vi "Dashboard Main.vi"() -> ()   [LabVIEW 2020]
uses:
  Support/Utility/FP_Size VI to Decoration Simple.vi/TypeDefs_Utility/Cluster_FP Set.ctl
  Support/Utility/FP_Size VI to Decoration Simple.vi/TypeDefs_Utility/ENUM RB_Pos_Quadrant Position.ctl
  <vilib>/event_ctls.llb/eventvkey.ctl
  a666340f-301f-4806-b1ce-2e5969000446.vi
  58c67c19-ca0f-4a2d-b08c-13e7632b1952.vi
  <vilib>/Rock Robotics/Network Tables/NT Read Numeric Array.vi
  <vilib>/Rock Robotics/WPI/Dashboard/WPI_DashboardLogging Global.vi
panel:
  out "Color 2":u32(colorbox)
  in  "Balance Speed":dbl=10.0 min=1.0 max=16.0 step=0.1 format="%.1g"
  out "RIO":string
  out "blink":bool
  out "Heartbeat":dbl
  out "Camera Image Right":T1(plugin-control)
  in  "Auto Select":string(combo)
  in  "Camera Settings Right":T2={"Frame Rate"=30, "Compression"=30, "Size"=1, "DB Camera Config"=FALSE} {"Frame Rate" scale=1.0..30.0; "Compression" scale=100.0..-1.0; "Size" items=["640x480", "320x240", "160x120"]}
  in  "Camera Name Right":string(combo)="No Camera Selection"
  out "Camera Perf":string
  in  "Camera Settings":T2={"Frame Rate"=30, "Compression"=30, "Size"=1, "DB Camera Config"=FALSE} {"Frame Rate" scale=1.0..30.0; "Compression" scale=100.0..-1.0; "Size" items=["640x480", "320x240", "160x120"]}
  in  "TCP":refnum<k5>
  in  "Rec Mode":enum32{"Stop", "Record", "Playback"}(radio)
  out "Robot IP":string
  out "Image Message":string="Timeout in Camera Communications"
  in  "Dashboard Tab":T3(tab)
  out "NT Connection":bool
  out "MotorChart R":cluster{"Numeric":dbl, "Numeric":dbl}(graph)
  out "MotorChart L":cluster{"Numeric":dbl, "Numeric":dbl}(graph)
  out "MotorSliders R":cluster{"MotorSlide1":dbl, "MotorSlide2":dbl} {"MotorSlide2" scale=-1.0..1.0 scale format="%#_2e"; "MotorSlide1" scale=-1.0..1.0 scale format="%#_2e"}
  out "MotorSliders L":cluster{"MotorSlide1":dbl, "MotorSlide2":dbl} {"MotorSlide2" scale=-1.0..1.0 scale format="%#_2e"; "MotorSlide1" scale=-1.0..1.0 scale format="%#_2e"}
  out "Gyro":dbl(knob) scale=0.0..360.0
  out "JS1 Z":dbl(slide) scale=-1.0..1.0 scale format="%#_2e"
  out "JS1 Graph":cluster{"X":dbl, "Y":dbl}[](graph)
  out "JS1 Buttons":T4
  out "JS2 Z":dbl(slide) scale=-1.0..1.0 scale format="%#_2e"
  out "JS2 Graph":cluster{"X":dbl, "Y":dbl}[](graph)
  out "JS2 Buttons":T4
  out "Mode":T5(ring)=enum."Auto Disabled"
  out "Right Camera Perf":cluster{"Bandwidth (Mbps)":dbl, "FPS":dbl}
  in  "DB/String 9":string
  in  "DB/String 8":string
  in  "DB/String 7":string
  in  "DB/String 6":string
  in  "DB/String 5":string
  in  "DB/String 4":string
  in  "DB/String 3":string
  in  "DB/String 2":string
  in  "DB/String 1":string
  in  "DB/String 0":string
  in  "DB/Slider 0":dbl(slide) scale=0.0..5.0
  in  "DB/Slider 1":dbl(slide) scale=0.0..5.0
  in  "DB/Slider 2":dbl(slide) scale=0.0..5.0
  in  "DB/Slider 3":dbl(slide) scale=0.0..5.0
  out "DB/LED 3":bool
  out "DB/LED 2":bool
  out "DB/LED 1":bool
  out "DB/LED 0":bool
  in  "DB/Button 3":bool
  in  "DB/Button 2":bool
  in  "DB/Button 1":bool
  in  "DB/Button 0":bool caption="New Name"
  in  "Test Slider":dbl(slide) scale=0.0..100.0 scale format="%#_3g"
  in  "On/Off":bool caption="Solenoid"
  in  "Test Name":u16(ring) items=["Select the test to run..."]
  in  "Test Tree":string(tree)
  in  "Motor":cluster{"Value":dbl, "Enable":bool} {"Value" scale=-1.0..1.0 scale format="%#_3g"}
  out "Progress":T6 {"Test Progress" scale=0.0..100.0}
  in  "Rev/Fwd":cluster{"Forward":bool, "Reverse":bool}
  in  "Test Ring":u16(ring) items=["Monochrome", "Color"]
  in  "CheckList":i32(listbox)
  out "Tree":string(tree)
  out "Camera Image":T1(plugin-control)
  in  "Camera Name":string(combo)="No Camera Selection"
  # "HW"
  # "HW"
  # "Joysticks"
  # "Drive Motors"
  # "Front"
  # "Right"
  # "Left"
  # "Back"
  # "This tab is a great place for autonomous settings and robot-specific values.\nPlace controls and indicators inside this tab and match name to\nDashboard Variables on robot. You can also delete this comment."
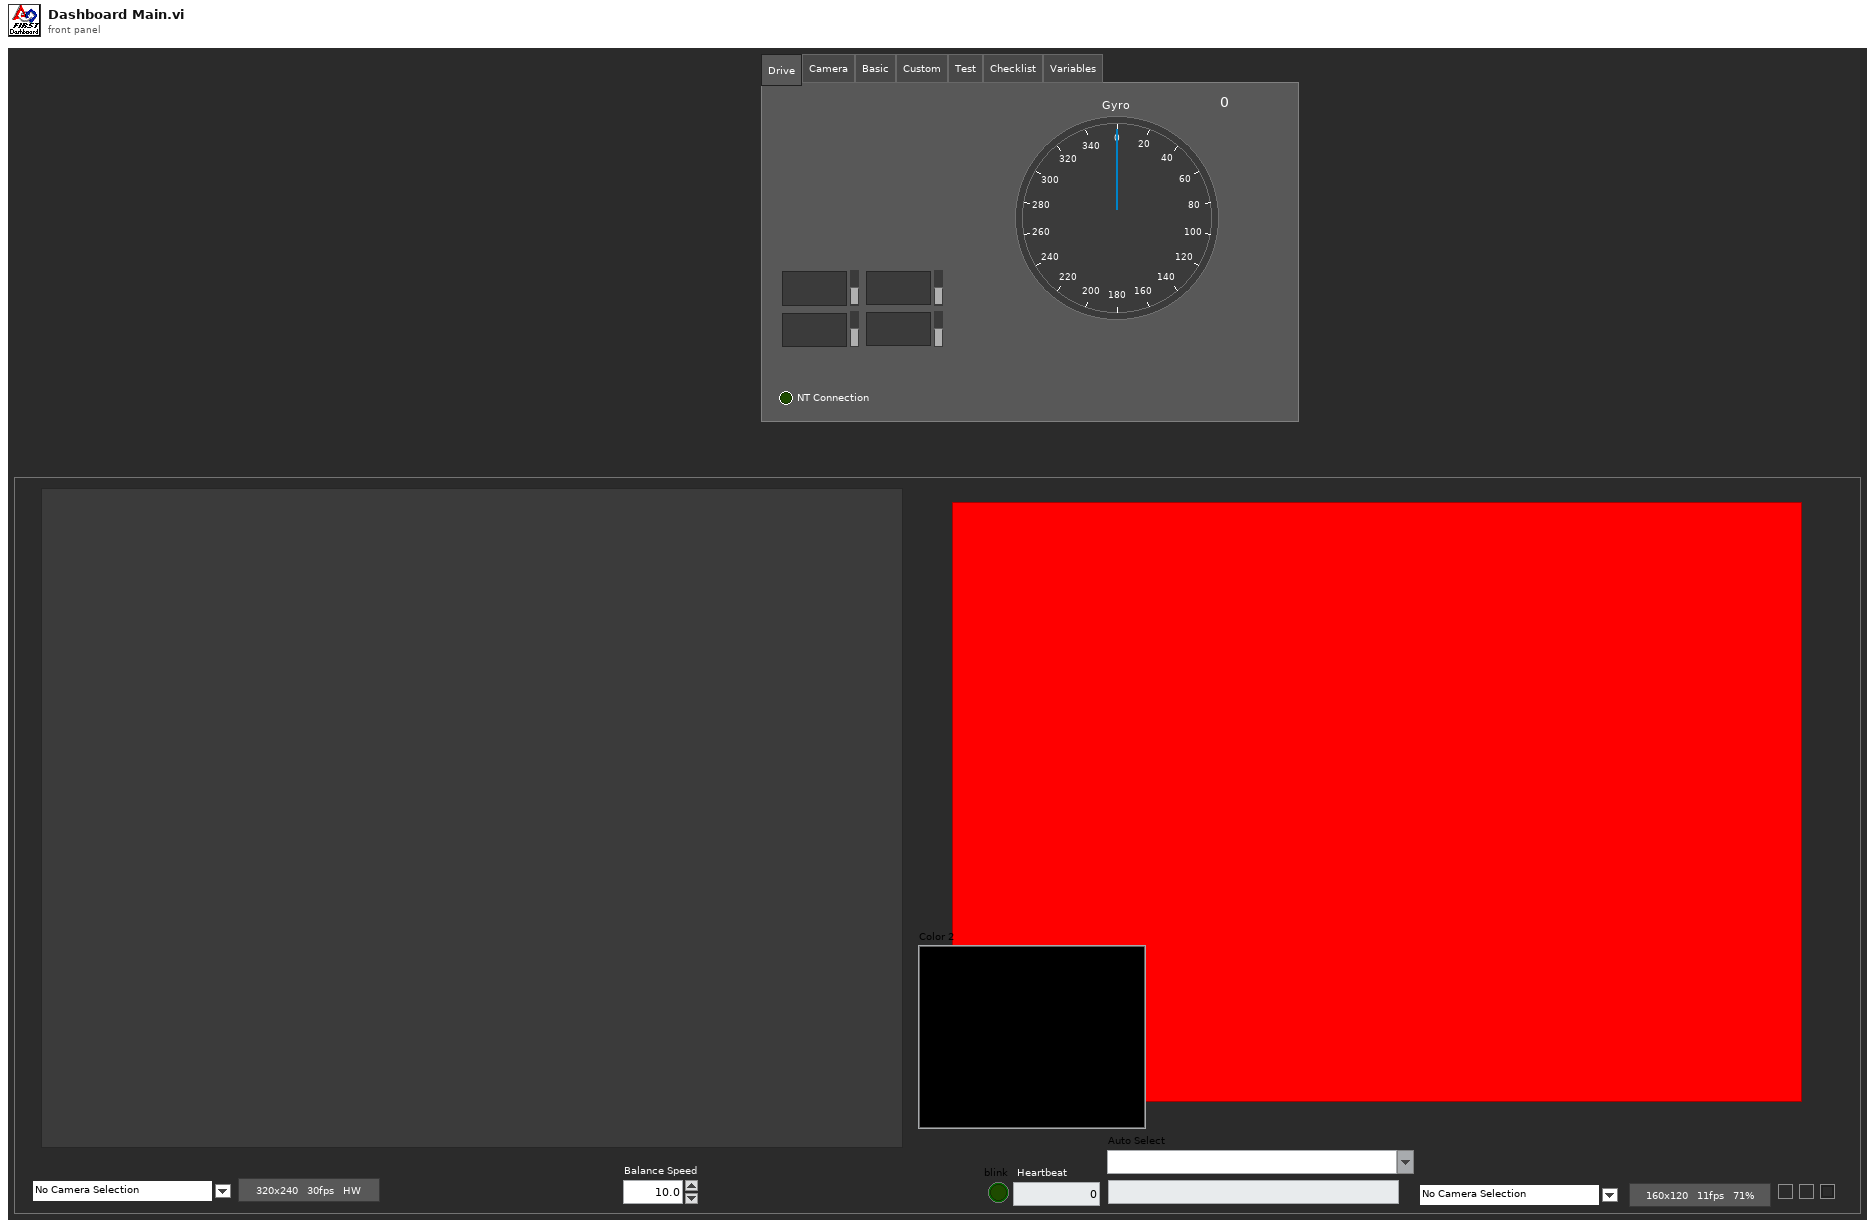
[diagram p1: front panel]
types:
  T1 = typedef "IMAQ Image.ctl" = refnum<image>
  T2 = cluster{"Frame Rate":i32, "Compression":i32, "Size":u16, "DB Camera Config":bool}
  T3 = enum32{"Drive", "Camera", "Basic", "Custom", "Test", "Checklist", "Variables"}
  T4 = cluster{bool, bool, bool, bool, bool, bool, bool, bool, bool, bool, bool, bool}
  T5 = enum8{"Tele-Op Disabled", "Tele-Op Enabled", "Auto Disabled", "Auto Enabled", "Test Disabled", "Test Enabled", "Disconnected", "No Code", "E-Stop"}
  T6 = cluster{"Test Progress":u8, "Test Progress Text":string}
  T7 = cluster{"Save Path":path, "Interval (s)":dbl, "Keep":i32}
  T8 = enum32{"Drive", "Camera", "Basic", "Custom", "Test", "Commands", "Checklist", "Variables"}
  T9 = typedef "Image Type" = u32
  T10 = cluster{"Error Strings":string, "Disable Counts":cluster{u16, u16}, "Rail Faults":cluster{u16, u16, u16}, "Robot IP":string, "DB Mode":u8, "Event Info":cluster{"Name":string, "Type":u8, "Number":u16, "Replay":u8}}
  T11 = cluster{"Storage":cluster{"Disk Free":u64, "RAM Block":u32, "RAM free":u32}, "CPU Utilization":cluster{"CPU % ISR":sgl, "CPU % Time Crit":sgl, "CPU % Timed Str":sgl, "CPU % High":sgl, "CPU % Above":sgl, "CPU % Normal":sgl, "CPU % Low":sgl}, "CAN":cluster{"% Bus Utilization":sgl, "Bus Off Cnt":u32, "TX_FIFO Full Cnt":u32, "Receive Error Cnt":u8, "Transmit Error Cnt":u8}, "HID":cluster{"HID Outputs":u32, "Rumble Low":u16, "Rumble High":u16}[]}
  T12 = cluster{"Status bits":cluster{"Test Mode":bool, "Autonomous":bool, "Enabled":bool, "Code Start":bool, "Brownout":bool, "Reserved 2":bool, "Reserved 3":bool, "E-Stop":bool}, "Code Trace":cluster{"Disabled":bool, "TeleOp":bool, "Auto":bool, "Test":bool}, "Controller Type":enum16{"unknown", "cRIO", "roboRio"}, "Code?":enum16{"unknown", "noCode", "code"}, "Battery V":dbl}
  T13 = cluster{"Control Bits":cluster{"TestMode":bool, "Autonomous":bool, "Enabled":bool, "FMS Present":bool, bool, bool, bool, "E-Stop":bool}, "Team Station ":u8, "Countdown":sgl, "Joystick Values":cluster{"Axes":dbl[], "Buttons":bool[], "POVs":i16[]}[]}
  T14 = cluster{"Axes":dbl[], "Buttons":bool[], "POVs":i16[]}[]
  T15 = cluster{"Axes":dbl[], "Buttons":bool[], "POVs":i16[]}
  T16 = cluster{"Buttons[0]":bool, "Buttons[1]":bool, "Buttons[2]":bool, "Buttons[3]":bool, "Buttons[4]":bool, "Buttons[5]":bool, "Buttons[6]":bool, "Buttons[7]":bool, "Buttons[8]":bool, "Buttons[9]":bool, "Buttons[10]":bool, "Buttons[11]":bool}
  T17 = typedef "Cluster_FP Set.ctl" = cluster{"Menu Bar":bool, "Position":T18, "Decoration index":i32, "border(px)":i32, "Monitor #":i32}
  T18 = typedef "ENUM RB_Pos_Quadrant Position.ctl" = enum32{"LFT-TOP", "MID-TOP", "RGT-TOP", "LFT-CTR", "MID-CTR", "RGT-CTR", "LFT-BOT", "MID-BOT", "RGT-BOT"}
  T19 = cluster{"Camera Image":refnum<vi>, "Tab":refnum<vi>, "Tab Button":refnum<vi>, "Rec Mode":refnum<vi>, "Test Slide":refnum<vi>, "Test On/Off":refnum<vi>, "Test Ring":refnum<vi>, "Test R/F":refnum<vi>, "Test Name":refnum<vi>, "Motor":refnum<vi>, "Progress":refnum<vi>, "LstBox Refnum":refnum<vi>, "Test Tree":refnum<vi>, "VblTree":refnum<vi>, "Camera Settings":refnum<vi>, "Camera Name":refnum<vi>, "perf info":refnum<vi>, "Camera Settings 2":refnum<vi>, "Camera Name 2":refnum<vi>, "Image Right":refnum<vi>}
  T20 = cluster{"Global Rectangle":i32[], "Contours":cluster{"Contour Type":u32, "ROI Type":u32, "Points":i32[]}[]}
  T21 = cluster{"Camera Name":string, string, "Saved DB Images Info":cluster{"Save Path":path, "Interval (s)":dbl, "Keep":i32}}
  T22 = cluster{"Camera Name Right":string, string, "Saved DB Images Info":cluster{"Save Path":path, "Interval (s)":dbl, "Keep":i32}}
  T23 = cluster{"Operation":enum16{"Update", "Clear"}, "Color Box":u32}[]
  T24 = typedef "eventvkey.ctl" = enum16{"ASCII", "Enter", "Return", "Shift", "Ctrl", "Alt", "Cmd", "Opt", "Caps", "NumLock", "Clear", "Break", "Up", "Down", "Left", "Right", "Insert", "Delete", "Home", "End", "PageUp", "PageDown", "Escape", "Help", "Pause", "ScrollLock", "F1", "F2", "F3", "F4", "F5", "F6", "F7", "F8", "F9", "F10", "F11", "F12", "F13", "F14", "F15", "F16", "F17", "F18", "F19", "F20", "F21", "F22", "F23", "F24", "Play", "VolumeUp", "VolumeDown", "Mute", "Two Byte Char"}
  T25 = cluster{"Image Size":bool, "Image Type":bool, "Pixel Value":bool, "ROI Information":bool, "Zoom Factor":bool}
  T26 = cluster{"Operation":enum16{"Update", "Clear"}, "Color Box":u32}
  T27 = cluster{"Shift":bool, "Ctrl":bool, "Alt":bool, "Cmd":bool, "Opt":bool}
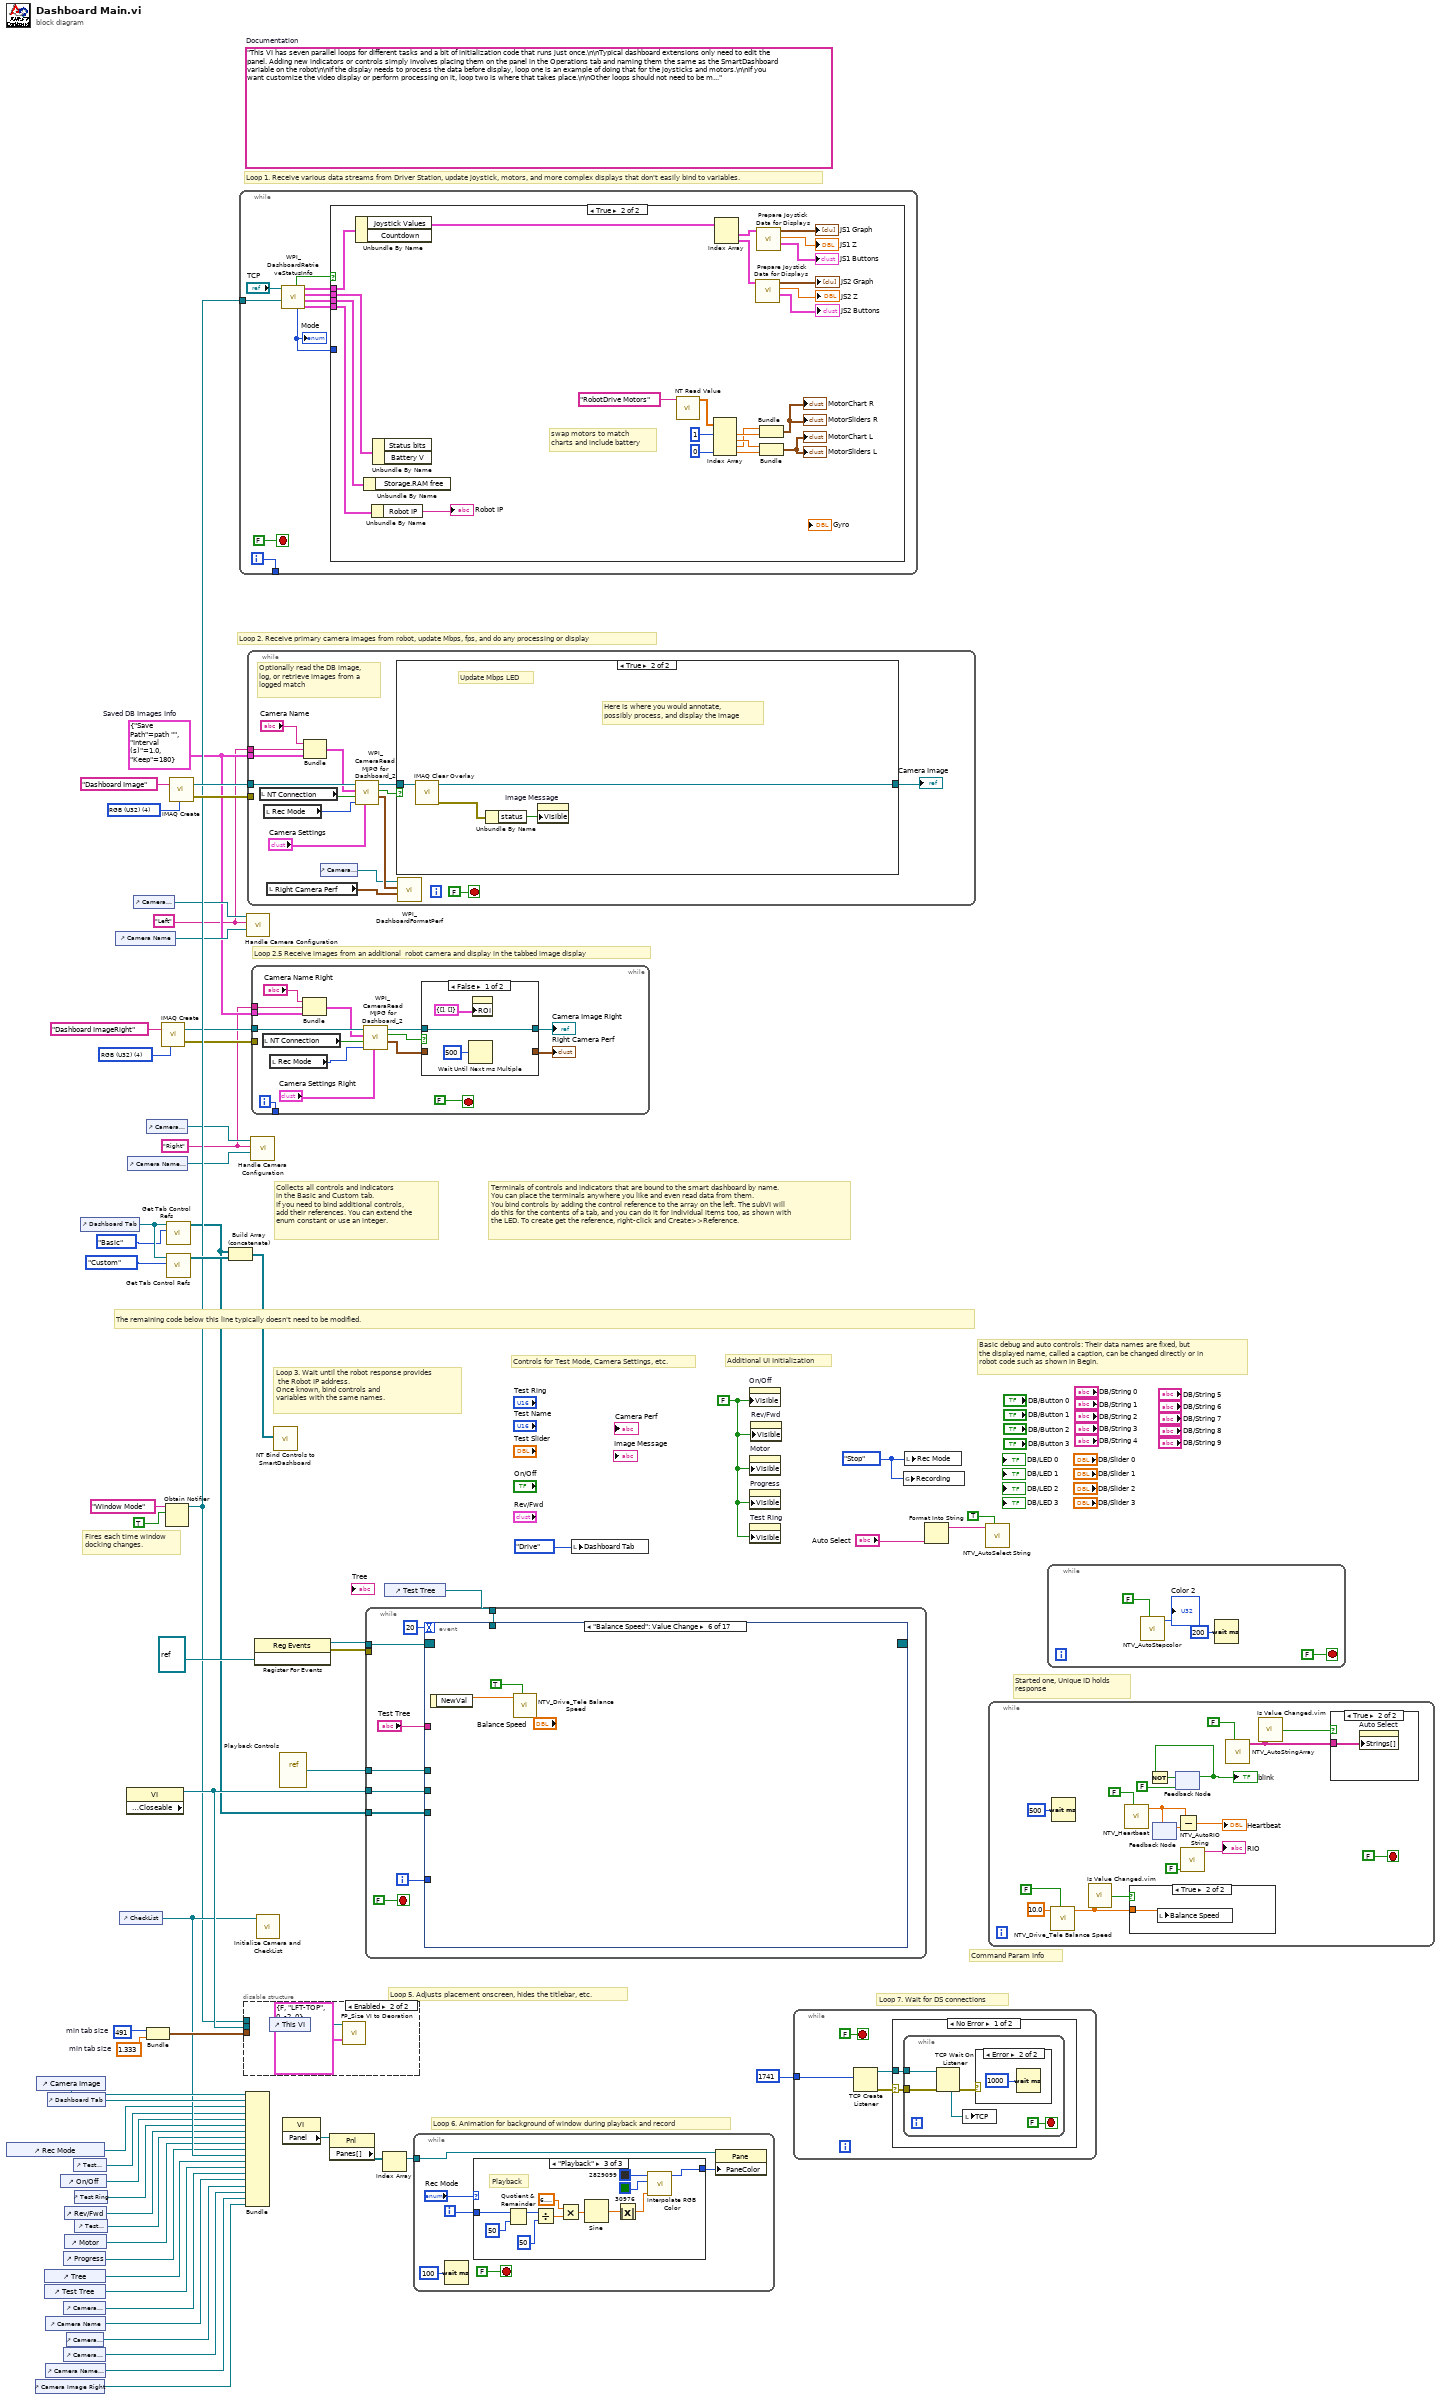
[diagram p0: block diagram]
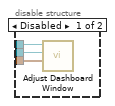
[diagram p4: hidden frame]
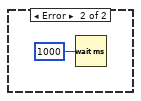
[diagram p7: hidden frame]
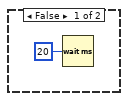
[diagram p8: hidden frame]
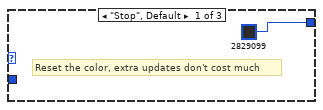
[diagram p9: hidden frame]
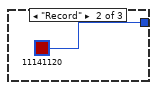
[diagram p10: hidden frame]
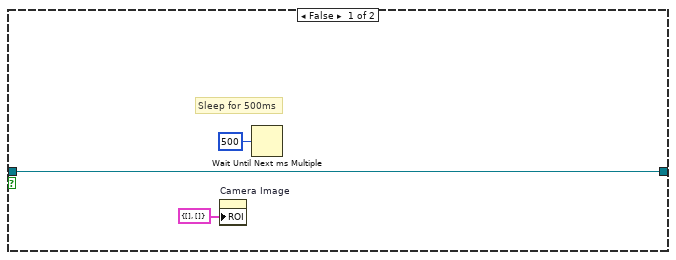
[diagram p11: hidden frame]
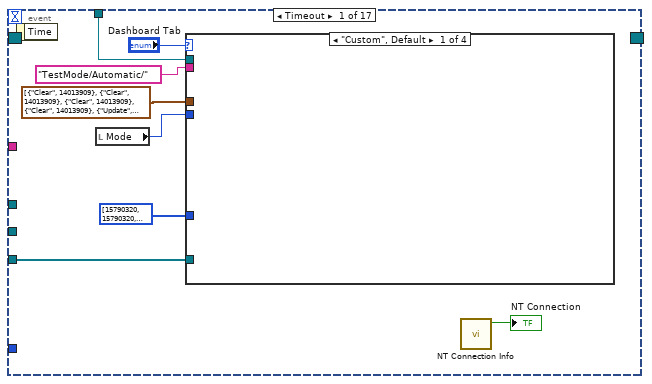
[diagram p12: hidden frame]
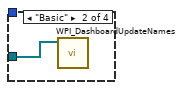
[diagram p13: hidden frame]
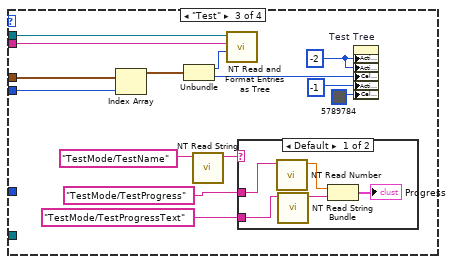
[diagram p14: hidden frame]
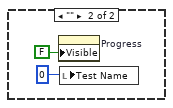
[diagram p15: hidden frame]
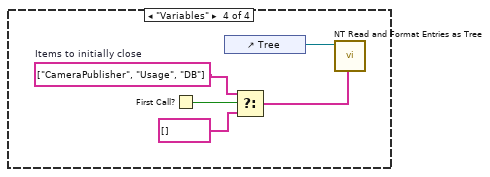
[diagram p16: hidden frame]
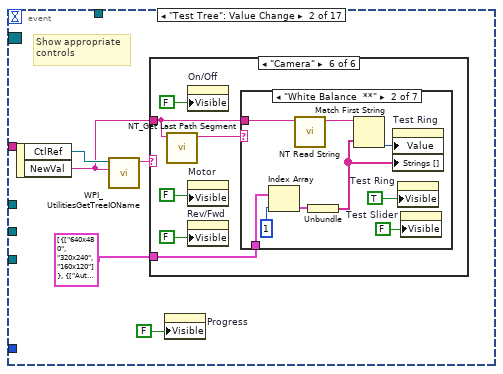
[diagram p17: hidden frame]
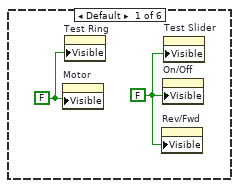
[diagram p18: hidden frame]
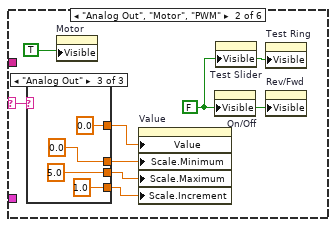
[diagram p19: hidden frame]
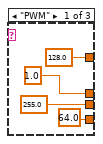
[diagram p20: hidden frame]
diagram:
  w6 = T7 {"Save Path"=path "", "Interval (s)"=1.0, "Keep"=180}  # Saved DB Images Info
  w5 = "Right"
  w4 = "Left"
  w16 = T9 4 items=["Grayscale (U8)", "Grayscale (I16)", "Grayscale (SGL)", "Complex (CSG)", "RGB (U32)", "HSL (U32)", "RGB (U64)"] ("Image Type")
  w41 = 491  # min tab size
  w40 = 1.333  # min tab size
  w48 = enum32{"Stop", "Record", "Playback"}."Stop" ("Rec Mode")
  w27 = FALSE ("Visible")
  (unwired) "This VI has seven parallel loops for different tasks and a bit of initialization code that runs just once.\n\nTypical dashboard extensions only need to edit the panel. Adding new indicators or controls simply involves placing them on the panel in the Operations tab and naming them the same as the SmartDashboard variable on the robot\n\nIf the display needs to process the data before display, loop one is an example of doing that for the joysticks and motors.\n\nIf you want customize the video display or perform processing on it, loop two is where that takes place.\n\nOther loops should not need to be modified. They are pretty standard, and document the task they perform."  # Documentation
  w62 = T9 4 items=["Grayscale (U8)", "Grayscale (I16)", "Grayscale (SGL)", "Complex (CSG)", "RGB (U32)", "HSL (U32)", "RGB (U64)"] ("Image Type")
  # "Loop 2.5 Receive images from an additional  robot camera and display in the tabbed image display"
  # "Command Param Info"
  # "Started one, Unique ID holds\nresponse"
  # "Loop 7. Wait for DS connections"
  # "Basic debug and auto controls: Their data names are fixed, but\nthe displayed name, called a caption, can be changed directly or in\nrobot code such as shown in Begin."
  # "Controls for Test Mode, Camera Settings, etc."
  # "Additional UI Initialization"
  # "Loop 6. Animation for background of window during playback and record"
  # "Fires each time window\ndocking changes."
  # "Collects all controls and indicators\nin the Basic and Custom tab.\nIf you need to bind additional controls,\nadd their references. You can extend the\nenum constant or use an integer."
  # "The remaining code below this line typically doesn't need to be modified."
  # "Terminals of controls and indicators that are bound to the smart dashboard by name.\nYou can place the terminals anywhere you like and even read data from them.\nYou bind controls by adding the control reference to the array on the left. The subVI will\ndo this for the contents of a tab, and you can do it for individual items too, as shown with\nthe LED. To create get the reference, right-click and Create>>Reference."
  # "Loop 3. Wait until the robot response provides\n the Robot IP address.\nOnce known, bind controls and\nvariables with the same names."
  # "Loop 5. Adjusts placement onscreen, hides the titlebar, etc."
  # "Loop 1. Receive various data streams from Driver Station, update joystick, motors, and more complex displays that don't easily bind to variables."
  # "Loop 2. Receive primary camera images from robot, update Mbps, fps, and do any processing or display"
  n1 = control-ref of="Rec Mode"() -> (w33:refnum<vi>)
  n2 = control-ref of="Camera Image Right"() -> (w9:refnum<vi>)
  n3 = control-ref of="Camera Image"() -> (w43:refnum<vi>)
  n4 = control-ref of="Tree"() -> (w37:refnum<vi>)
  n5 = control-ref of="Test Tree"() -> (w36:refnum<vi>)
  n6 = control-ref of="Camera Name"() -> (w20:refnum<vi>)
  n7 = control-ref of="Camera Name Right"() -> (w10:refnum<vi>)
  n8 = control-ref of="Dashboard Tab"() -> (w42:refnum<vi>)
  n9 = control-ref of="On/Off"() -> (w31:refnum<vi>)
  n10 = control-ref of="Progress"() -> (w28:refnum<vi>)
  n11 = control-ref of="Camera Settings"() -> (w21:refnum<vi>)
  n12 = control-ref of="Camera Settings Right"() -> (w11:refnum<vi>)
  n13 = control-ref of="Rev/Fwd"() -> (w29:refnum<vi>)
  n14 = control-ref of="Motor"() -> (w34:refnum<vi>)
  n15 = control-ref of="Camera Perf"() -> (w19:refnum<vi>)
  n16 = control-ref of="Test Slider"() -> (w32:refnum<vi>)
  n17 = control-ref of="Test Ring"() -> (w30:refnum<vi>)
  n18 = control-ref of="Test Name"() -> (w35:refnum<vi>)
  n19 = control-ref of="Dashboard Tab"() -> (w46:refnum<vi>)
  n20 = control-ref of="Camera Name"() -> (w22:refnum<vi>)
  n21 = control-ref of="CheckList"() -> (w38:refnum<vi>)
  n22 = property class="VI" props=["Front Panel.Closeable"]() -> (reference out=w47:refnum<vi>)  [unwired: 2 in, 2 out]
  n23 = control-ref of="Camera Name Right"() -> (w12:refnum<vi>)
  n24 = control-ref of="Camera Settings"() -> (w23:refnum<vi>)
  n25 = control-ref of="Camera Settings Right"() -> (w13:refnum<vi>)
  n26 = Bundle("min tab size"=w41, "min tab size"=w40) -> (w39:cluster{"min tab size":i32, "min tab size":dbl})  [unwired: 1 in]
  n27 = call "IMAQ Create"("Image Name"="Dashboard ImageRight", "Image Type"=w16) -> ("New Image"=w15:T1, "error out"=w14:errorcluster)  [unwired: 2 in, 1 out]
  n28 = Obtain Notifier(name (unnamed)="Window Mode", notification data type=TRUE) -> (notifier out=w26:refnum<notifier>)  [unwired: 2 in, 2 out]
  n29 = call <vilib>:"Get Tab Control Refs.vi"("Page Index"=T8."Basic" ("Dashboard Tab"), "TabControl in"=w46) -> ("ControlsOnPage"=w18:refnum<vi>[])  [unwired: 9 in]
  n30 = call <vilib>:"Get Tab Control Refs.vi"("Page Index"=T8."Custom" ("Dashboard Tab"), "TabControl in"=w46) -> ("ControlsOnPage"=w45:refnum<vi>[])  [unwired: 9 in]
  n31 = call "IMAQ Create"("Image Name"="Dashboard Image", "Image Type"=w62) -> ("New Image"=w60:T1, "error out"=w59:errorcluster)  [unwired: 2 in, 1 out]
  n32 = Build Array (concatenate)(w18, w45) -> (w44:refnum<vi>[])
  n33 = while {
    tunnel: [w71] -> _
    tunnel: w26 -> [w63]
    i -> [w71]
    stop <- FALSE stop-if-true
    n34 = call <vilib>:"WPI_DashboardRetrieveStatusInfo.vi"("Window Mode Notifier"=w63, "TCP Cnx"="TCP") -> ("Power and Errors"=w66:T10, "Robot Metrics"=w69:T11, "Status Info"=w70:T12, "Control Info"=w67:T13, "Robot Mode"=w65:T5, "Process?"=w68:bool)  [unwired: 4 in]
    "Mode" <- w65
    n35 = case shown="True" w68 {
      tunnel: w70 -> [_ w97]
      tunnel: w69 -> [_ w96]
      tunnel: w67 -> [_ w95]
      tunnel: w66 -> [_ w94]
      tunnel: w65 -> [_ _]
      frame False {
        n36 = Wait (ms)(milliseconds to wait=u32 20) -> ()  [unwired: 1 out]
      }
      frame True {
        # "swap motors to match\ncharts and include battery"
        n37 = Unbundle By Name(w95) -> ("Joystick Values"=w85:T14)  [unwired: 1 out]
        n38 = Unbundle By Name(w96) -> ()  [unwired: 1 out]
        n39 = Unbundle By Name(w94) -> ("Robot IP"=→"Robot IP":string)
        n40 = Unbundle By Name(w97) -> ()  [unwired: 2 out]
        n41 = call-poly <vilib>:"NT Read Value.vi"("name"="RobotDrive Motors" ("Name")) -> ("value"=w75:dbl[])  [unwired: 8 in, 2 out]
        n42 = Index Array(array=w75, index #1=1, index #4=0) -> (element #1=w89:dbl, element #2=w90:dbl, element #3=w88:dbl, element #4=w93:dbl)  [unwired: 2 in]
        n43 = Index Array(array=w85) -> (element #1=w84:T15, element #2=w80:T15)  [unwired: 2 in]
        n44 = call "Prepare Joystick Data for Displays.vi"("Joystick Values"=w80) -> ("Buttons"=→"JS2 Buttons":T16, "Z Axis"=→"JS2 Z":dbl, "Cartesian Data"=→"JS2 Graph":cluster{"X axis":dbl, "X axis":dbl}[])  [unwired: 8 in]
        n45 = call "Prepare Joystick Data for Displays.vi"("Joystick Values"=w84) -> ("Buttons"=→"JS1 Buttons":T16, "Z Axis"=→"JS1 Z":dbl, "Cartesian Data"=→"JS1 Graph":cluster{"X axis":dbl, "X axis":dbl}[])  [unwired: 8 in]
        n46 = Bundle("Numeric"=w88, "Numeric"=w89) -> (→"MotorChart R" →"MotorSliders R":cluster{"Numeric":dbl, "Numeric":dbl})  [unwired: 1 in]
        n47 = Bundle("Numeric"=w90, "Numeric"=w93) -> (→"MotorChart L" →"MotorSliders L":cluster{"Numeric":dbl, "Numeric":dbl})  [unwired: 1 in]
      }
    }
  }
  n48 = disable-structure shown="Enabled" {
    disable-tunnel: w47 -> [w101 _]
    disable-tunnel: w39 -> [w100 _]
    disable-tunnel: w26 -> [w98 _]
    frame Disabled {
      n49 = call "Adjust Dashboard Window.vi"("Size Constraints"=w100, "VI"=w101, "WIn Mode"=w98) -> ("Sizing Refnums"=w99:T19)  [unwired: 8 in]
    }
    frame Enabled {
      n50 = control-ref of="This VI"() -> (w103:refnum<vi>)
      n51 = call "FP_Size VI to Deoration.vi"("FPSet"=T17 {"Menu Bar"=FALSE, "Position"=enum."LFT-TOP", "Decoration index"=0, "border(px)"=-2, "Monitor #"=0}, "VI Ref"=w103) -> ()  [unwired: 8 in, 2 out]
    }
  }
  n52 = Bundle("Camera Image"=w43, "Dashboard Tab"=w42, "Rec Mode"=w33, "Test Slider"=w32, "On/Off"=w31, "Test Ring"=w30, "Rev/Fwd"=w29, "Test Name"=w35, "Motor"=w34, "Progress"=w28, "CheckList"=w38, "Tree"=w37, "Test Tree"=w36, "Camera Settings"=w21, "Camera Name"=w20, "Camera Perf"=w19, "Camera Settings Right"=w11, "Camera Name Right"=w10, "Camera Image Right"=w9) -> ()  [unwired: 1 in, 1 out]
  n53 = call "Handle Camera Configuration.vi"("CameraNameRef"=w22, "Display Name"=w4, "ClusterRef"=w23) -> ()  [unwired: 9 in]
  n54 = while {
    tunnel: w60 -> [w117]
    tunnel: w59 -> [_]
    tunnel: w6 -> [w110]
    tunnel: w4 -> [w107]
    stop <- FALSE stop-if-true
    # "Optionally read the DB image,\nlog, or retrieve images from a\nlogged match"
    n55 = local read "NT Connection"() -> (w111:bool)
    n56 = local read "Rec Mode"() -> (w114:enum32{"Stop", "Record", "Playback"})
    n57 = local read "Right Camera Perf"() -> (w105:cluster{"Bandwidth (Mbps)":dbl, "FPS":dbl})
    n58 = Bundle("Camera Name"="Camera Name", w107, "Saved DB Images Info"=w110) -> (w109:T21)  [unwired: 1 in]
    n59 = control-ref of="Camera Perf"() -> (w104:refnum<vi>)
    n60 = call <vilib>:"WPI_CameraRead MJPG for Dashboard_2.vi"("Camera Settings"="Camera Settings", "Rec Mode"=w114, "NT Connection"=w111, "Capture Info"=w109, "Image in"=w117) -> ("perf info"=w106:cluster{"Bandwidth (Mbps)":dbl, "fps":dbl}, "Active"=w115:bool, "Image\\ out"=w116:T1)  [unwired: 4 in]
    n61 = case shown="True" w115 {
      tunnel: w116 -> [w120 w123]
      tunnel: [w120 w122] -> w112
      frame False {
        # "Sleep for 500ms"
        n62 = property on="Camera Image" class="ImageControl"("ROI"=T20 {"Global Rectangle"=[], "Contours"=[]}) -> ()  [unwired: 2 in, 2 out]
        n63 = Wait Until Next ms Multiple(millisecond multiple=u32 500) -> ()  [unwired: 1 out]
      }
      frame True {
        # "Here is where you would annotate,\npossibly process, and display the image"
        # "Update Mbps LED"
        n64 = call "IMAQ Clear Overlay"("Image"=w123) -> ("error out"=w124:errorcluster, "Image Out"=w122:T1)  [unwired: 2 in, 7 out]
        n65 = Unbundle By Name(w124) -> ("status"=w125:bool)
        n66 = property on="Image Message" class="Str"("Visible"=w125) -> ()  [unwired: 2 in, 2 out]
      }
    }
    "Camera Image" <- w112
    n67 = call <vilib>:"WPI_DashboardFormatPerf.vi"("Right Camera Perf"=w105, "Performance"=w106, "String in"=w104) -> ()  [unwired: 9 in]
  }
  n68 = call "Handle Camera Configuration.vi"("CameraNameRef"=w12, "Display Name"=w5, "ClusterRef"=w13) -> ()  [unwired: 9 in]
  n69 = while {
    tunnel: w15 -> [w140]
    tunnel: w14 -> [_]
    tunnel: [w135] -> _
    tunnel: w6 -> [w131]
    tunnel: w5 -> [w128]
    i -> [w135]
    stop <- FALSE stop-if-true
    n70 = local read "NT Connection"() -> (w132:bool)
    n71 = local read "Rec Mode"() -> (w139:enum32{"Stop", "Record", "Playback"})
    n72 = Bundle("Camera Name Right"="Camera Name Right", w128, "Saved DB Images Info"=w131) -> (w130:T22)  [unwired: 1 in]
    n73 = call <vilib>:"WPI_CameraRead MJPG for Dashboard_2.vi"("Camera Settings"="Camera Settings Right", "Rec Mode"=w139, "NT Connection"=w132, "Capture Info"=w130, "Image in"=w140) -> ("perf info"=w126:cluster{"Bandwidth (Mbps)":dbl, "fps":dbl}, "Active"=w134:bool, "Image\\ out"=w137:T1)  [unwired: 4 in]
    n74 = case shown="False" w134 {
      tunnel: w137 -> [w142 w145]
      tunnel: [w142 w145] -> w133
      tunnel: [_ w144] -> w127
      tunnel: w126 -> [_ w144]
      frame False {
        n75 = Wait Until Next ms Multiple(millisecond multiple=u32 500) -> ()  [unwired: 1 out]
        n76 = property on="Camera Image Right" class="ImageControl"("ROI"=T20 {"Global Rectangle"=[], "Contours"=[]}) -> ()  [unwired: 2 in, 2 out]
      }
      frame True {
      }
    }
    "Camera Image Right" <- w133
    "Right Camera Perf" <- w127
  }
  n77 = register-events(refnum<vi> refnum) -> (reference out=w51:refnum<event-registration>, error out=w50:errorcluster)  [unwired: 2 in]
  n78 = call "Initialize Camera and CheckList.vi"("ListBox in"=w38) -> ()  [unwired: 11 in]
  n79 = call <vilib>:"NT Bind Controls to SmartDashboard.vi"("Bound Control Refs"=w44) -> ()  [unwired: 11 in]
  n80 = vi-ref "Playback Controls.vi"() -> (w52:refnum<vi>)
  n81 = property class="VI"() -> ("Panel"=w54:refnum<vi>)  [unwired: 2 in, 2 out]
  n82 = property class="Pnl"(reference=w54) -> ("Panes[]"=w55:refnum<vi>[])  [unwired: 1 in, 2 out]
  n83 = Index Array(array=w55) -> (element=w53:refnum<vi>)  [unwired: 1 in]
  n84 = control-ref of="Test Tree"() -> (w56:refnum<vi>)
  n85 = while {
    tunnel: w56 -> [w152]
    tunnel: w52 -> [w151]
    tunnel: w51 -> [w150]
    tunnel: w50 -> [_]
    tunnel: w47 -> [w149]
    tunnel: w18 -> [w148]
    i -> [w146]
    stop <- FALSE stop-if-true
    n86 = event shown="[5] \"Balance Speed\": Value Change" {
      selector: w150 -> [_ _ _ _ _ _ _ _ _ _ _ _ _ _ _ _ _]
      dyn-events: [_ _ _ _ _ _ _ _ _ _ _ _ _ w356 _ _ _] -> _
      timeout: 20 -> [_ _ _ _ _ _ _ _ _ _ _ _ _ _ _ _ _]
      tunnel: w152 -> [w161 _ _ _ _ _ _ _ _ _ _ _ _ _ _ _ _]
      tunnel: "Test Tree" -> [_ _ _ _ _ _ _ _ w329 w336 w337 w340 w347 _ _ _ _]
      tunnel: w151 -> [_ _ _ _ _ _ _ _ _ _ _ _ _ w358 _ w373 _]
      tunnel: w149 -> [_ _ _ _ _ _ _ _ _ _ _ _ _ w354 _ _ _]
      tunnel: w148 -> [w156 _ _ _ _ _ _ _ _ _ _ _ _ _ _ _ _]
      tunnel: w146 -> [_ _ _ _ _ _ _ _ _ _ _ _ _ _ _ _ _]
      event Timeout {
        n87 = event-data() -> ()  [unwired: 1 in, 1 out]
        n88 = local read "Mode"() -> (w159:T5)
        n89 = case shown="\"Custom\", Default" "Dashboard Tab" {
          tunnel: w161 -> [_ _ w177 _]
          tunnel: "TestMode/Automatic/" ("Name Pattern") -> [_ _ w176 _]
          tunnel: T23 [{"Operation"=enum."Clear", "Color Box"=14013909}, {"Operation"=enum."Clear", "Color Box"=14013909}, {"Operation"=enum."Clear", "Color Box"=14013909}, {"Operation"=enum."Clear", "Color Box"=14013909}, {"Operation"=enum."Update", "Color Box"=14013909}, {"Operation"=enum."Update", "Color Box"=16777215}, {"Operation"=enum."Clear", "Color Box"=14013909}, {"Operation"=enum."Clear", "Color Box"=14013909}, {"Operation"=enum."Clear", "Color Box"=14013909}] -> [_ _ w169 _]
          tunnel: w159 -> [_ _ w168 _]
          tunnel: u32[] [15790320, 15790320, 15790320, 15790320, 16777215, 16777215, 15790320, 15790320, 15790320] -> [_ _ _ _]
          tunnel: w156 -> [_ w163 _ _]
          frame "Custom", Default {
          }
          frame "Basic" {
            n90 = call <vilib>:"WPI_DashboardUpdateNames.vi"("Controls on Tab"=w163) -> ()  [unwired: 11 in]
          }
          frame "Test" {
            w175 = -2 ("Active Item:Row Number")
            n91 = Index Array(array=w169, index=w168) -> (element=w170:T26)
            n92 = Unbundle(w170) -> ("Operation"=w171:enum16{"Update", "Clear"}, "Color Box"=w172:u32)
            n93 = call <vilib>:"NT Read String.vi"("name"="TestMode/TestName" ("Name")) -> ("value"=w166:string)  [unwired: 8 in, 2 out]
            n94 = call <vilib>:"NT Read and Format Entries as Tree.vi"("Operation"=w171, "Name Pattern"=w176, "Tree Refnum"=w177) -> ()  [unwired: 7 in, 2 out]
            n95 = case shown="Default" w166 {
              tunnel: "TestMode/TestProgress" ("Name") -> [w179 _]
              tunnel: "TestMode/TestProgressText" ("Name") -> [w178 _]
              frame Default {
                n96 = call <vilib>:"NT Read Number.vi"("name"=w179) -> ("value"=w180:dbl)  [unwired: 8 in, 2 out]
                n97 = call <vilib>:"NT Read String.vi"("name"=w178) -> ("value"=w181:string)  [unwired: 8 in, 2 out]
                n98 = Bundle("value"=w180, "value"=w181) -> (→"Progress":cluster{"value":dbl, "value":string})  [unwired: 1 in]
              }
              frame "" {
                n99 = property on="Progress" class="Clust (strict)"("Visible"=FALSE) -> ()  [unwired: 2 in, 2 out]
                n100 = local write "Test Name"(u16 0) -> ()
              }
            }
            n101 = property on="Test Tree" class="Tree (strict)"("Active Item Row Number"=w175, "ActiveColNum"=w175, "CellBG"=w172, "Active Item Row Number"=-1 ("Active Item:Row Number"), "CellBG"=u32 5789784 ("Color Box")) -> ()  [unwired: 2 in, 2 out]
          }
          frame "Variables" {
            w187 = string[] ["CameraPublisher", "Usage", "DB"]  # Items to initially close
            n102 = First Call?() -> (First Call?: T/F=w188:bool)
            n103 = control-ref of="Tree"() -> (w189:refnum<vi>)
            n104 = Select(t=w187, s=w188, f=string[] []) -> (s? t:f=w185:string[])
            n105 = call <vilib>:"NT Read and Format Entries as Tree.vi"("Tags to  Close"=w185, "Tree Refnum"=w189) -> ()  [unwired: 8 in, 2 out]
          }
        }
        n106 = call <vilib>:"NT Connection Info.vi"() -> ("Connected"=→"NT Connection":bool)  [unwired: 11 in]
      }
      event "Test Tree": Value Change {
        # "Show appropriate\ncontrols"
        n107 = event-data() -> ("CtlRef"=w193:refnum<vi>, "NewVal"=w191:string)  [unwired: 1 in]
        n108 = call <vilib>:"WPI_UtilitiesGetTreeIOName.vi"("NewVal"=w191, "TreeControl in"=w193) -> ("I/O Name"=w194:string)  [unwired: 9 in]
        n109 = case shown="\"Camera\"" w194 {
          selector: w194 -> [_ w201 _ w223 w232 _]
          tunnel: w191 -> [_ _ w220 w222 _ w239]
          tunnel: cluster{string[]}[] [{["640x480", "320x240", "160x120"]}, {["Auto", "Fixed indoor", "Fixed outdoor 1", "Fixed outdoor 2", "Fixed fluorescent 1", "Fixed fluorescent 2", "Hold current"]}, {["Auto", "Flicker-free 50 Hz", "Flicker-free 60 Hz", "Hold current"]}, {["None", "Prioritize frame rate", "Prioritize image quality"]}, {["Monochrome", "Color"]}] -> [_ _ _ _ _ w238]
          frame Default {
            w196 = FALSE ("Visible")
            w195 = FALSE ("Visible")
            n110 = property on="Motor" class="Clust (strict)"("Visible"=w195) -> ()  [unwired: 2 in, 2 out]
            n111 = property on="Test Ring" class="Ring (strict)"("Visible"=w195) -> ()  [unwired: 2 in, 2 out]
            n112 = property on="Rev/Fwd" class="Clust (strict)"("Visible"=w196) -> ()  [unwired: 2 in, 2 out]
            n113 = property on="On/Off" class="Bool (strict)"("Visible"=w196) -> ()  [unwired: 2 in, 2 out]
            n114 = property on="Test Slider" class="Slide (strict)"("Visible"=w196) -> ()  [unwired: 2 in, 2 out]
          }
          frame "Analog Out", "Motor", "PWM" {
            w202 = FALSE ("Visible")
            n115 = case shown="\"Analog Out\"" w201 {
              tunnel: [1.0 ("Value") -1.0 ("Value") 0.0 ("Value")] -> w200
              tunnel: [255.0 ("Value") 1.0 ("Value") 5.0 ("Value")] -> w199
              tunnel: [128.0 ("Value") 0.0 ("Value") 0.0 ("Value")] -> w198
              tunnel: [64.0 ("Value") 0.5 ("Value") 1.0 ("Value")] -> w197
              frame "PWM" {
              }
              frame "Motor", Default {
              }
              frame "Analog Out" {
              }
            }
            n116 = property on="Motor" class="Clust (strict)"("Visible"=TRUE) -> ()  [unwired: 2 in, 2 out]
            n117 = property on="Value" class="Slide (strict)"("Value"=w198, "Scale.Minimum"=w200, "Scale.Maximum"=w199, "Scale.Increment"=w197) -> ()  [unwired: 2 in, 2 out]
            n118 = property on="On/Off" class="Bool (strict)"("Visible"=w202) -> ()  [unwired: 2 in, 2 out]
            n119 = property on="Test Slider" class="Slide (strict)"("Visible"=w202) -> ()  [unwired: 2 in, 2 out]
            n120 = property on="Test Ring" class="Ring (strict)"("Visible"=w202) -> ()  [unwired: 2 in, 2 out]
            n121 = property on="Rev/Fwd" class="Clust (strict)"("Visible"=w202) -> ()  [unwired: 2 in, 2 out]
          }
          frame "Servo" {
            w218 = FALSE ("Visible")
            n122 = call <vilib>:"NT Read Number.vi"("name"=w220) -> ("value"=w219:dbl)  [unwired: 8 in, 2 out]
            n123 = property on="Test Slider" class="Slide (strict)"("Visible"=TRUE, "Scale.Maximum"=170.0 ("Scale.Range:Maximum")) -> ()  [unwired: 2 in, 2 out]
            n124 = local write "Test Slider"(w219) -> ()
            n125 = property on="Motor" class="Clust (strict)"("Visible"=w218) -> ()  [unwired: 2 in, 2 out]
            n126 = property on="Rev/Fwd" class="Clust (strict)"("Visible"=w218) -> ()  [unwired: 2 in, 2 out]
            n127 = property on="On/Off" class="Bool (strict)"("Visible"=w218) -> ()  [unwired: 2 in, 2 out]
            n128 = property on="Test Ring" class="Ring (strict)"("Visible"=w218) -> ()  [unwired: 2 in, 2 out]
          }
          frame "Relay", "Solenoid" {
            w221 = FALSE ("Visible")
            n129 = property on="Motor" class="Clust (strict)"("Visible"=w221) -> ()  [unwired: 2 in, 2 out]
            n130 = property on="Test Slider" class="Slide (strict)"("Visible"=w221) -> ()  [unwired: 2 in, 2 out]
            n131 = Search and Replace String(input string=w222, search string="/Value  **", replace string="/Direction") -> (result string=w228:string)  [unwired: 5 in, 3 out]
            n132 = property on="Test Ring" class="Ring (strict)"("Visible"=w221) -> ()  [unwired: 2 in, 2 out]
            n133 = call <vilib>:"NT Read String.vi"("name"=w228) -> ("value"=w226:string)  [unwired: 8 in, 2 out]
            n134 = Equal?(x="Both directions", y=w226) -> (x = y?=w224:bool)
            n135 = Not(x=w224) -> (.not. x?=w225:bool)
            n136 = property on="Rev/Fwd" class="Clust (strict)"("Visible"=w224) -> ()  [unwired: 2 in, 2 out]
            n137 = property on="On/Off" class="Bool (strict)"("Visible"=w225, "Caption.Text"=w223) -> ()  [unwired: 2 in, 2 out]
          }
          frame "Compressor", "Digital Out" {
            w231 = FALSE ("Visible")
            # "Get direction and finish"
            n138 = property on="Motor" class="Clust (strict)"("Visible"=w231) -> ()  [unwired: 2 in, 2 out]
            n139 = property on="Test Slider" class="Slide (strict)"("Visible"=w231) -> ()  [unwired: 2 in, 2 out]
            n140 = property on="Test Ring" class="Ring (strict)"("Visible"=w231) -> ()  [unwired: 2 in, 2 out]
            n141 = property on="On/Off" class="Bool (strict)"("Visible"=TRUE, "Caption.Text"=w232) -> ()  [unwired: 2 in, 2 out]
            n142 = property on="Rev/Fwd" class="Clust (strict)"("Visible"=FALSE) -> ()  [unwired: 2 in, 2 out]
          }
          frame "Camera" {
            n143 = call <vilib>:"NT_Get Last Path Segment.vi"("String in"=w239) -> ("String out"=w240:string)  [unwired: 10 in]
            n144 = property on="On/Off" class="Bool (strict)"("Visible"=FALSE) -> ()  [unwired: 2 in, 2 out]
            n145 = property on="Motor" class="Clust (strict)"("Visible"=FALSE) -> ()  [unwired: 2 in, 2 out]
            n146 = property on="Rev/Fwd" class="Clust (strict)"("Visible"=FALSE) -> ()  [unwired: 2 in, 2 out]
            n147 = case shown="\"White Balance  **\"" w240 {
              tunnel: w239 -> [w246 w255 w264 w273 w282 _ w288]
              tunnel: w238 -> [w244 w252 w261 w270 w279 _ _]
              frame "Size  **" {
                n148 = Index Array(array=w244) -> (element=w243:cluster{string[]})  [unwired: 1 in]
                n149 = call <vilib>:"NT Read String.vi"("name"=w246) -> ("value"=w245:string)  [unwired: 8 in, 2 out]
                n150 = Unbundle(w243) -> (w241:string[])
                n151 = Match First String(2:w241, 3:w245) -> (0:w242:i32)  [unwired: 1 out]
                n152 = property on="Test Ring" class="Ring (strict)"("Value"=w242, "Strings []"=w241) -> ()  [unwired: 2 in, 2 out]
                n153 = property on="Test Ring" class="Ring (strict)"("Visible"=TRUE) -> ()  [unwired: 2 in, 2 out]
                n154 = property on="Test Slider" class="Slide (strict)"("Visible"=FALSE) -> ()  [unwired: 2 in, 2 out]
              }
              frame "White Balance  **" {
                n155 = Index Array(array=w252, index=1) -> (element=w253:cluster{string[]})
                n156 = call <vilib>:"NT Read String.vi"("name"=w255) -> ("value"=w254:string)  [unwired: 8 in, 2 out]
                n157 = Unbundle(w253) -> (w250:string[])
                n158 = Match First String(2:w250, 3:w254) -> (0:w249:i32)  [unwired: 1 out]
                n159 = property on="Test Ring" class="Ring (strict)"("Value"=w249, "Strings []"=w250) -> ()  [unwired: 2 in, 2 out]
                n160 = property on="Test Ring" class="Ring (strict)"("Visible"=TRUE) -> ()  [unwired: 2 in, 2 out]
                n161 = property on="Test Slider" class="Slide (strict)"("Visible"=FALSE) -> ()  [unwired: 2 in, 2 out]
              }
              frame "Exposure  **" {
                n162 = Index Array(array=w261, index=2) -> (element=w262:cluster{string[]})
                n163 = call <vilib>:"NT Read String.vi"("name"=w264) -> ("value"=w263:string)  [unwired: 8 in, 2 out]
                n164 = Unbundle(w262) -> (w258:string[])
                n165 = Match First String(2:w258, 3:w263) -> (0:w259:i32)  [unwired: 1 out]
                n166 = property on="Test Ring" class="Ring (strict)"("Value"=w259, "Strings []"=w258) -> ()  [unwired: 2 in, 2 out]
                n167 = property on="Test Ring" class="Ring (strict)"("Visible"=TRUE) -> ()  [unwired: 2 in, 2 out]
                n168 = property on="Test Slider" class="Slide (strict)"("Visible"=FALSE) -> ()  [unwired: 2 in, 2 out]
              }
              frame "Exposure Priority  **" {
                n169 = Index Array(array=w270, index=3) -> (element=w271:cluster{string[]})
                n170 = call <vilib>:"NT Read String.vi"("name"=w273) -> ("value"=w272:string)  [unwired: 8 in, 2 out]
                n171 = Unbundle(w271) -> (w267:string[])
                n172 = Match First String(2:w267, 3:w272) -> (0:w268:i32)  [unwired: 1 out]
                n173 = property on="Test Ring" class="Ring (strict)"("Value"=w268, "Strings []"=w267) -> ()  [unwired: 2 in, 2 out]
                n174 = property on="Test Ring" class="Ring (strict)"("Visible"=TRUE) -> ()  [unwired: 2 in, 2 out]
                n175 = property on="Test Slider" class="Slide (strict)"("Visible"=FALSE) -> ()  [unwired: 2 in, 2 out]
              }
              frame "Color Enable  **" {
                n176 = Index Array(array=w279, index=4) -> (element=w280:cluster{string[]})
                n177 = call <vilib>:"NT Read String.vi"("name"=w282) -> ("value"=w281:string)  [unwired: 8 in, 2 out]
                n178 = Unbundle(w280) -> (w276:string[])
                n179 = Match First String(2:w276, 3:w281) -> (0:w277:i32)  [unwired: 1 out]
                n180 = property on="Test Ring" class="Ring (strict)"("Value"=w277, "Strings []"=w276) -> ()  [unwired: 2 in, 2 out]
                n181 = property on="Test Ring" class="Ring (strict)"("Visible"=TRUE) -> ()  [unwired: 2 in, 2 out]
                n182 = property on="Test Slider" class="Slide (strict)"("Visible"=FALSE) -> ()  [unwired: 2 in, 2 out]
              }
              frame Default {
                n183 = property on="Test Ring" class="Ring (strict)"("Visible"=FALSE) -> ()  [unwired: 2 in, 2 out]
                n184 = property on="Test Slider" class="Slide (strict)"("Visible"=FALSE) -> ()  [unwired: 2 in, 2 out]
              }
              frame "Brightness  **", "Color Level  **", "Compression  **", "FPS  **", "Sharpness  **" {
                n185 = call <vilib>:"NT Read Number.vi"("name"=w288) -> ("value"=w287:dbl)  [unwired: 8 in, 2 out]
                n186 = local write "Test Slider"(w287) -> ()
                n187 = property on="Test Slider" class="Slide (strict)"("Visible"=TRUE, "Scale.Maximum"=100.0 ("Scale.Range:Maximum")) -> ()  [unwired: 2 in, 2 out]
                n188 = property on="Test Ring" class="Ring (strict)"("Visible"=FALSE) -> ()  [unwired: 2 in, 2 out]
              }
            }
          }
        }
        n189 = property on="Progress" class="Clust (strict)"("Visible"=FALSE) -> ()  [unwired: 2 in, 2 out]
      }
      event "Test Name": Mouse Enter {
        # "Populate the ring with the list of tests"
        n190 = event-data() -> ()  [unwired: 1 in, 1 out]
        n191 = call <vilib>:"NT Read String Array.vi"("name"="TestMode/TestList" ("Name")) -> ("value"=w295:string[])  [unwired: 8 in, 2 out]
        n192 = Build Array (concatenate)("Select the test to run...", w295) -> (w294:string[])
        n193 = property on="Test Name" class="Ring (strict)"("Strings []"=w294) -> ()  [unwired: 2 in, 2 out]
      }
      event "Test Name": Value Change {
        w296 = FALSE ("Visible")
        # "Tell the robot the test name to run"
        n194 = event-data() -> ("NewVal"=w300:u16)  [unwired: 1 in]
        n195 = property on="Test Name" class="Ring (strict)"() -> ("Strings []"=w301:string[])  [unwired: 2 in, 2 out]
        n196 = local write "Progress"(T6 {"Test Progress"=0, "Test Progress Text"=""} ("Progress")) -> ()
        n197 = Index Array(array=w301, index=w300) -> (element=w299:string)
        n198 = call <vilib>:"NT Write String.vi"("value"=w299, "name"="TestMode/TestName" ("Name")) -> ()  [unwired: 9 in, 1 out]
        n199 = property on="Progress" class="Clust (strict)"("Visible"=TRUE) -> ()  [unwired: 2 in, 2 out]
        n200 = property on="Motor" class="Clust (strict)"("Visible"=w296) -> ()  [unwired: 2 in, 2 out]
        n201 = property on="Test Slider" class="Slide (strict)"("Visible"=w296) -> ()  [unwired: 2 in, 2 out]
        n202 = property on="On/Off" class="Bool (strict)"("Visible"=w296) -> ()  [unwired: 2 in, 2 out]
        n203 = property on="Rev/Fwd" class="Clust (strict)"("Visible"=w296) -> ()  [unwired: 2 in, 2 out]
        n204 = property on="Test Ring" class="Ring (strict)"("Visible"=w296) -> ()  [unwired: 2 in, 2 out]
      }
      event "Auto Select": Value Change {
        n205 = event-data() -> ("NewVal"=w303:string)  [unwired: 1 in]
        n206 = call "NTV_AutoSelect String.vi"("Read(f) Write(t)"=TRUE, "Auto RIO"=w303) -> ()  [unwired: 9 in, 1 out]
      }
      event "Balance Speed": Value Change {
        n207 = event-data() -> ("NewVal"=w306:dbl)  [unwired: 1 in]
        n208 = call "NTV_Drive_Tele Balance Speed.vi"("Read(f) Write(t)"=TRUE, "Balance Speed"=w306) -> ()  [unwired: 9 in, 1 out]
      }
      event "CheckList": Double Click {
        # "Shift clears all"
        # "Update symbols on the listbox"
        n209 = event-data() -> ("PlatMods.Shift"=w307:bool, "Row"=w309:i32)  [unwired: 1 in]
        n210 = case shown="True" w307 {
          tunnel: w309 -> [w313 _]
          tunnel: 1 -> [w312 _]
          frame False {
            n211 = property on="CheckList" class="LstBox (strict)"() -> ("Item Symbols"=w311:i32[])  [unwired: 2 in, 2 out]
            n212 = Replace Array Subset(array=w311, new element=w312, index=w313) -> (w310:i32[])
            n213 = property on="CheckList" class="LstBox (strict)"("Item Symbols"=w310) -> ()  [unwired: 2 in, 2 out]
          }
          frame True {
            w314 = 0 ("Top Row")
            n214 = property on="CheckList" class="LstBox (strict)"() -> ("Number of Rows"=w316:u32)  [unwired: 2 in, 2 out]
            n215 = Initialize Array(0, w316) -> (w315:i32[])
            n216 = property on="CheckList" class="LstBox (strict)"("Top Row"=w314, "Value"=w314, "Item Symbols"=w315) -> ()  [unwired: 2 in, 2 out]
          }
        }
      }
      event "CheckList": Key Down {
        # "Update symbols on the listbox\nLeft and right keys check and uncheck"
        n217 = event-data() -> ("VKey"=w319:T24)  [unwired: 1 in]
        n218 = case shown="\"Left\", \"Right\"" w319 {
          selector: w319 -> [w324 _]
          tunnel: eventvkey."Left" ("VKey") -> [w322 _]
          frame "Left", "Right" {
            n219 = Equal?(x=w322, y=w324) -> (x = y?=w323:bool)
            n220 = Select(t=0, s=w323, f=1) -> (s? t:f=w325:i32)
            n221 = property on="CheckList" class="LstBox (strict)"() -> ("Item Symbols"=w328:i32[])  [unwired: 2 in, 2 out]
            n222 = Replace Array Subset(array=w328, new element=w325, index="CheckList") -> (w327:i32[])
            n223 = property on="CheckList" class="LstBox (strict)"("Item Symbols"=w327) -> ()  [unwired: 2 in, 2 out]
          }
          frame Default {
          }
        }
      }
      event "Motor.Enable": Value Change {
        # "When the test mode otor enable helper is set, update that\ntree row item's value"
        n224 = event-data() -> ("NewVal"=w333:bool)  [unwired: 1 in]
        n225 = Unbundle("Motor") -> ("Value"=w332:dbl)  [unwired: 1 out]
        n226 = Select(t=w332, s=w333, f=0.0) -> (s? t:f=w330:dbl)
        n227 = call <vilib>:"NT Write Number.vi"("value"=w330, "name"=w329) -> ()  [unwired: 9 in, 1 out]
      }
      event "Test Slider": Value Change {
        # "When the test mode slider helper is set, update that\ntree row item's value"
        n228 = event-data() -> ("NewVal"=w335:dbl)  [unwired: 1 in]
        n229 = call <vilib>:"NT Write Number.vi"("value"=w335, "name"=w336) -> ()  [unwired: 9 in, 1 out]
      }
      event "On/Off": Value Change {
        # "When the test mode on/off helper value is set, update that\ntree row item's value"
        n230 = event-data() -> ("NewVal"=w339:bool)  [unwired: 1 in]
        n231 = Boolean To (0,1)(Boolean=w339) -> (0, 1=w338:i16)
        n232 = call <vilib>:"NT Write Number.vi"("value"=w338, "name"=w337) -> ()  [unwired: 9 in, 1 out]
      }
      event "Rev/Fwd": Value Change {
        # "When the test mode helper value for relays is set, update that\ntree row item's value"
        n233 = event-data() -> ("NewVal.Forward"=w346:bool, "NewVal.Reverse"=w345:bool)  [unwired: 1 in]
        n234 = Boolean To (0,1)(Boolean=w346) -> (0, 1=w342:i16)
        n235 = Boolean To (0,1)(Boolean=w345) -> (0, 1=w344:i16)
        n236 = Negate(x=w344) -> (-x=w343:i16)
        n237 = Add(x=w342, y=w343) -> (x+y=w341:i16)
        n238 = call <vilib>:"NT Write Number.vi"("value"=w341, "name"=w340) -> ()  [unwired: 9 in, 1 out]
      }
      event "Test Ring": Value Change {
        # "When a test mode helper value is selected from the ring,\nset the tree item's variable to the string value"
        n239 = event-data() -> ("NewVal"=w349:u16)  [unwired: 1 in]
        n240 = property on="Test Ring" class="Ring (strict)"() -> ("Strings []"=w350:string[])  [unwired: 2 in, 2 out]
        n241 = Index Array(array=w350, index=w349) -> (element=w348:string)
        n242 = call <vilib>:"NT Write String.vi"("value"=w348, "name"=w347) -> ()  [unwired: 9 in, 1 out]
      }
      event "Rec Mode": Value Change {
        # "Update globals for recording mode and path to read log from.\nClear when logging and let NetworkTables set path for vision to\nuse."
        n243 = event-data() -> ("NewVal"=w359:enum32{"Stop", "Record", "Playback"})  [unwired: 1 in]
        n244 = global write "WPI_DashboardLogging Global.vi" "Logging Filename"(path "") -> ()
        n245 = global write "WPI_DashboardLogging Global.vi" "Recording"(w359) -> ()
        n246 = case shown="\"Playback\"" w359 {
          tunnel: w358 -> [_ w361 w369]
          tunnel: [_ _ w368] -> w356
          tunnel: [_ _ w367] -> _
          tunnel: w354 -> [_ _ w365]
          tunnel: cluster{i32, i32} {-250, 170} -> [_ _ w364]
          tunnel: [_ _ T25 {"Image Size"=TRUE, "Image Type"=TRUE, "Pixel Value"=TRUE, "ROI Information"=TRUE, "Zoom Factor"=FALSE} ("Image Information Shown:All Elements")] -> w351
          tunnel: [_ _ TRUE ("Zoom Factor")] -> w352
          frame Default {
          }
          frame "Stop", "Record" {
            # "Place Window too"
            n247 = invoke class="VI" method="FP.Close"(reference=w361) -> (reference out=w360:refnum<vi>)  [unwired: 2 in, 2 out]
            n248 = invoke class="VI" method="Abort VI"(reference=w360) -> ()  [unwired: 2 in, 3 out]
          }
          frame "Playback" {
            n249 = call "Open Playback Panel.vi"("Offset"=w364, "DB VI Ref"=w365, "Playback in"=w369) -> ("Playback out"=w366:refnum<vi>)  [unwired: 8 in]
            n250 = register-events(w366) -> (reference out=w368:refnum<event-registration>, error out=w367:errorcluster)  [unwired: 2 in]
          }
        }
        n251 = property on="Camera Image Right" class="ImageControl"("Image Information Shown"=w351, "Image Information Visible"=w352) -> ()  [unwired: 2 in, 2 out]
        n252 = property on="Camera Image" class="ImageControl"("Image Information Shown"=w351, "Image Information Visible"=w352) -> ()  [unwired: 2 in, 2 out]
        n253 = call <vilib>:"WPI_DashboardNT Log FieldName Cache.vi"("Operation"=enum16{"Lookup/Add", "Index", "Clear"}."Clear") -> ()  [unwired: 8 in, 3 out]
      }
      event Panel Close {
        w370 = enum32{"Stop", "Record", "Playback"}."Stop" ("Rec Mode")
        # "Playback window has been closed, abort"
        n254 = event-data() -> ()  [unwired: 1 in, 4 out]
        n255 = local write "Rec Mode"(w370) -> ()
        n256 = global write "WPI_DashboardLogging Global.vi" "Recording"(w370) -> ()
      }
      event Panel Close {
        # "Abort playback window and ourself"
        n257 = event-data() -> ()  [unwired: 1 in, 4 out]
        n258 = invoke class="VI" method="FP.Close"(reference=w373) -> (reference out=w372:refnum<vi>)  [unwired: 2 in, 2 out]
        n259 = invoke class="VI" method="Abort VI"(reference=w372) -> (error out=w371:errorcluster)  [unwired: 2 in, 2 out]
        n260 = invoke class="VI" method="Abort VI"(error in=w371) -> ()  [unwired: 2 in, 3 out]
      }
      event "Tree": Double Click {
        n261 = event-data() -> ("PlatMods"=w379:T27, "Tag"=w376:string)  [unwired: 1 in]
        n262 = Unbundle(w379) -> ("Shift"=w378:bool)  [unwired: 4 out]
        n263 = String Subset(string=w376, length (rest)=1 ("length (rest)")) -> (substring=w375:string)  [unwired: 1 in]
        n264 = Not(x=w378) -> (.not. x?=w377:bool)
        n265 = case shown="\"/\"" w375 {
          tunnel: w376 -> [_ w381]
          tunnel: w377 -> [_ w380]
          frame Default {
          }
          frame "/" {
            n266 = call <vilib>:"NT Update Persistence.vi"("Persistence"=w380, "Name"=w381) -> ()  [unwired: 9 in, 1 out]
          }
        }
      }
    }
  }
  n267 = while {
    tunnel: w53 -> [w383]
    i -> [w386]
    stop <- FALSE stop-if-true
    n268 = Wait (ms)(milliseconds to wait=u32 100) -> ()  [unwired: 1 out]
    n269 = case shown="\"Playback\"" "Rec Mode" {
      tunnel: w386 -> [_ _ w401]
      tunnel: [u32 2829099 ("Base Color") u32 11141120 ("Target Color") w390] -> w382
      frame "Stop", Default {
        # "Reset the color, extra updates don't cost much"
      }
      frame "Record" {
      }
      frame "Playback" {
        # "Playback"
        n270 = Quotient & Remainder(x=w401, y=u32 50 ("milliseconds to wait")) -> (x-y*floor(x/y)=w397:u32)  [unwired: 1 out]
        n271 = Divide(x=w397, y=u32 50 ("milliseconds to wait")) -> (x/y=w394:dbl)
        n272 = Multiply(x=6.283185307179586, y=w394) -> (x*y=w399:dbl)
        n273 = Sine(x=w399) -> (sin(x)=w398:dbl)
        n274 = Absolute Value(x=w398) -> (abs(x)=w391:dbl)
        n275 = call "Interpolate RGB Color.vi"("Proportion"=w391, "Target Color"=u32 30976, "Base Color"=u32 2829099) -> ("Result Color"=w390:u32)  [unwired: 8 in]
      }
    }
    n276 = property class="Pane"(reference=w383, "PaneColor"=w382) -> ()  [unwired: 1 in, 2 out]
  }
  n277 = local write "Dashboard Tab"(T3."Drive" ("Dashboard Tab")) -> ()
  n278 = property on="On/Off" class="Bool (strict)"("Visible"=w27) -> ()  [unwired: 2 in, 2 out]
  n279 = property on="Motor" class="Clust (strict)"("Visible"=w27) -> ()  [unwired: 2 in, 2 out]
  n280 = property on="Progress" class="Clust (strict)"("Visible"=w27) -> ()  [unwired: 2 in, 2 out]
  n281 = property on="Test Ring" class="Ring (strict)"("Visible"=w27) -> ()  [unwired: 2 in, 2 out]
  n282 = property on="Rev/Fwd" class="Clust (strict)"("Visible"=w27) -> ()  [unwired: 2 in, 2 out]
  n283 = while {
    tunnel: u16 1741 ("timeout ms (25000)") -> [w403]
    stop <- FALSE stop-if-true
    n284 = TCP Create Listener(10:w403) -> (0:w402:errorcluster, 3:w404:refnum<k5>)  [unwired: 4 in, 1 out]
    n285 = case shown="No Error" w402 {
      selector: w402 -> [w406 _]
      tunnel: w404 -> [w407 _]
      frame No Error {
        n286 = while {
          tunnel: w407 -> [w410]
          tunnel: w406 -> [w409]
          stop <- FALSE stop-if-true
          n287 = TCP Wait On Listener(8:w409, 11:w410) -> (0:w411:errorcluster, 4:w412:refnum<k5>)  [unwired: 2 in, 3 out]
          n288 = local write "TCP"(w412) -> ()
          n289 = case shown="Error" w411 {
            frame No Error {
            }
            frame Error {
              n290 = Wait (ms)(milliseconds to wait=u32 1000) -> ()  [unwired: 1 out]
            }
          }
        }
      }
      frame Error {
        n291 = Wait (ms)(milliseconds to wait=u32 1000) -> ()  [unwired: 1 out]
      }
    }
  }
  n292 = global write "WPI_DashboardLogging Global.vi" "Recording"(w48) -> ()
  n293 = local write "Rec Mode"(w48) -> ()
  n294 = Format Into String("Auto Select") -> (resulting string=w2:string)  [unwired: 3 in, 1 out]
  n295 = call "NTV_AutoSelect String.vi"("Read(f) Write(t)"=TRUE, "Auto RIO"=w2) -> ()  [unwired: 9 in, 1 out]
  n296 = while {
    stop <- FALSE stop-if-true
    n297 = call "NTV_Drive_Tele Balance Speed.vi"("Read(f) Write(t)"=FALSE, "Balance Speed"=10.0) -> ("Balance Speed"=w416:dbl)  [unwired: 9 in]
    n298 = Wait (ms)(milliseconds to wait=u32 500) -> ()  [unwired: 1 out]
    n299 = call "Is Value Changed.vim"("value"=w416) -> ("changed or first call?"=w417:bool)
    n300 = call "NTV_Heartbeat.vi"("Read(f) Write(t)"=FALSE) -> ("Heartbeat"=w430:dbl)  [unwired: 10 in]
    n301 = case shown="True" w417 {
      tunnel: w416 -> [_ w433]
      frame False {
      }
      frame True {
        n302 = local write "Balance Speed"(w433) -> ()
      }
    }
    n303 = feedback #1() -> (w429:dbl)  [unwired: 1 in]
    n304 = feedback-in #1(w430) -> ()
    n305 = feedback #2(FALSE) -> (w425:bool)
    "blink" <- w425
    n306 = Not(x=w425) -> (.not. x?=w426:bool)
    n307 = feedback-in #2(w426) -> ()
    n308 = Subtract(x=w430, y=w429) -> (x-y=→"Heartbeat":dbl)
    n309 = call "NTV_AutoRIO String.vi"("Read(f) Write(t)"=FALSE) -> ("Auto RIO"=→"RIO":string)  [unwired: 10 in]
    n310 = call "NTV_AutoStringArray.vi"("Read(f) Write(t)"=FALSE) -> ("Array 2"=w422:string[])  [unwired: 10 in]
    n311 = call "Is Value Changed.vim"("value"=w422) -> ("changed or first call?"=w421:bool)
    n312 = case shown="True" w421 {
      tunnel: w422 -> [_ w434]
      frame False {
      }
      frame True {
        n313 = property on="Auto Select" class="CmbBox"("Strings[]"=w434) -> ()  [unwired: 2 in, 2 out]
      }
    }
  }
  n314 = while {
    stop <- FALSE stop-if-true
    n315 = call "NTV_AutoStepcolor.vi"("Read(f) Write(t)"=FALSE) -> ("Color 2"=→"Color 2":u32)  [unwired: 10 in]
    n316 = Wait (ms)(milliseconds to wait=u32 200) -> ()  [unwired: 1 out]
  }
